vi "Initialize.vi"(6 "Error In":errorcluster, 7 "Duration (s)":dbl=300.0, 8 "Buoy SE":T1 {"North" format="%#_10f"; "East" format="%#_8f"}, 9 "Buoy SW":T1 {"North" format="%#_10f"; "East" format="%#_8f"}, 10 "Buoy NE":T1 {"North" format="%#_10f"; "East" format="%#_8f"}, 11 "Buoy NW":T1 {"North" format="%#_10f"; "East" format="%#_8f"}) -> (0 "Error Out":errorcluster, 3 "StationKeeping out":refnum<class "StationKeeping.lvclass">)   [LabVIEW 2011, in "StationKeeping.lvclass"]
uses:
  StationKeeping.lvclass
  2 Typedefs/UTM Location.ctl
  StationKeeping.lvclass/StationKeeping.ctl
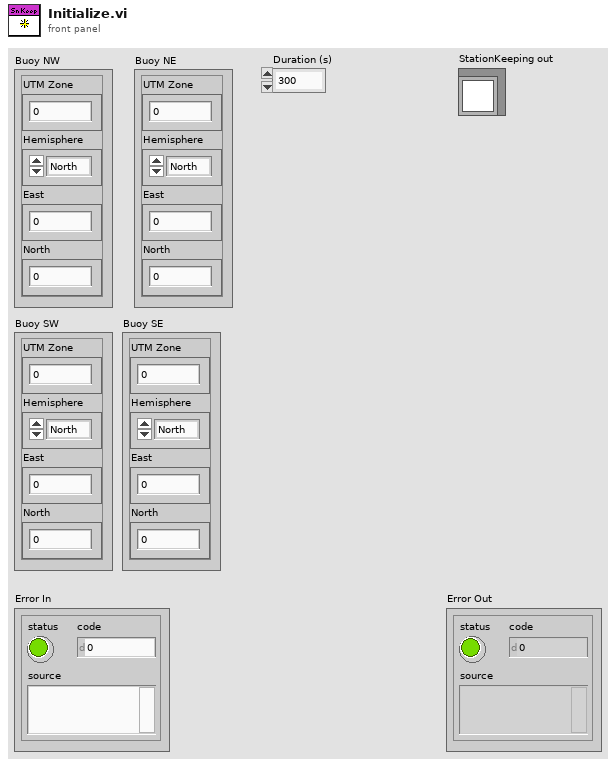
[diagram p1: front panel]
types:
  T1 = typedef "UTM Location.ctl" = cluster{"UTM Zone":dbl, "Hemisphere":enum16{"North", "South"}, "East":dbl, "North":dbl}
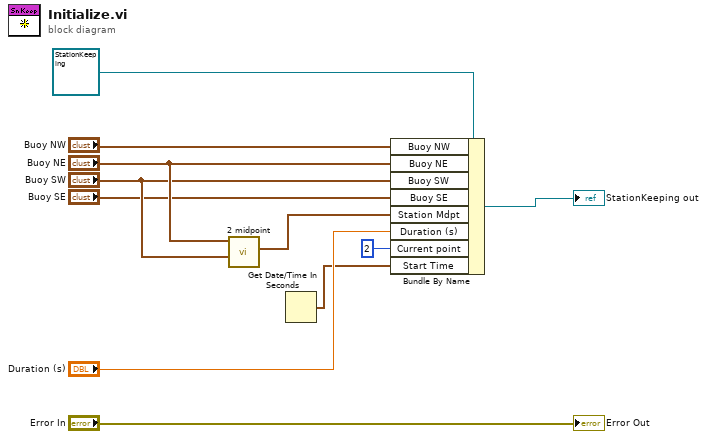
[diagram p0: block diagram]
diagram:
  n1 = call "2 midpoint.vi"("UTM 2"="Buoy SW", "UTM 1"="Buoy NE") -> ("Midpoint"=w5:T1)  [unwired: 8 in, 1 out]
  n2 = Get Date/Time In Seconds() -> (seconds since 1Jan1904=w1:timestamp)
  n3 = Bundle By Name(cluster=refnum<class "StationKeeping.lvclass"> refnum ("StationKeeping in"), "Buoy NW"="Buoy NW", "Buoy NE"="Buoy NE", "Buoy SW"="Buoy SW", "Buoy SE"="Buoy SE", "Station Mdpt"=w5, "Duration (s)"="Duration (s)", "Current point"=2, "Start Time"=w1) -> (→"StationKeeping out":refnum<class "StationKeeping.lvclass">)
  "Error Out" <- "Error In"
